vi "NOAH_jr.vi"() -> ()   [LabVIEW 2017]
panel:
  in  "Rates":dbl
  in  "Outliers":dbl
  in  "Max":dbl
  in  "Min":dbl
  in  "Range":dbl
  in  "Standard Deviation":dbl
  in  "Median":dbl
  in  "Mean":dbl
  in  "Data Source":string
  in  "Fault Text":string
  out "Posting Time":timestamp format="%<%H:%M:%S>T"
  out "Time to Handle":timestamp format="%<%H:%M:%S>T"
  out "Fault Priority Rank":dbl
  out "Notification Light":bool
  out "OK Time":timestamp format="%<%H:%M:%S>T"
  in  "Problem Count":dbl
  in  "Prompt Count":dbl
  in  "Warning Count":dbl
  in  "Total Notifications":dbl format="%#.0g"
  # "At-a-Glance"
  # "Fault Information"
  # "Priority"
  # "to handle"
  # "Posted at"
  # "Pinned Items"
  # "Analytics"
  # "Model HQ"
  # "Analytical"
  # "Grey-Box"
  # "Data-Driven"
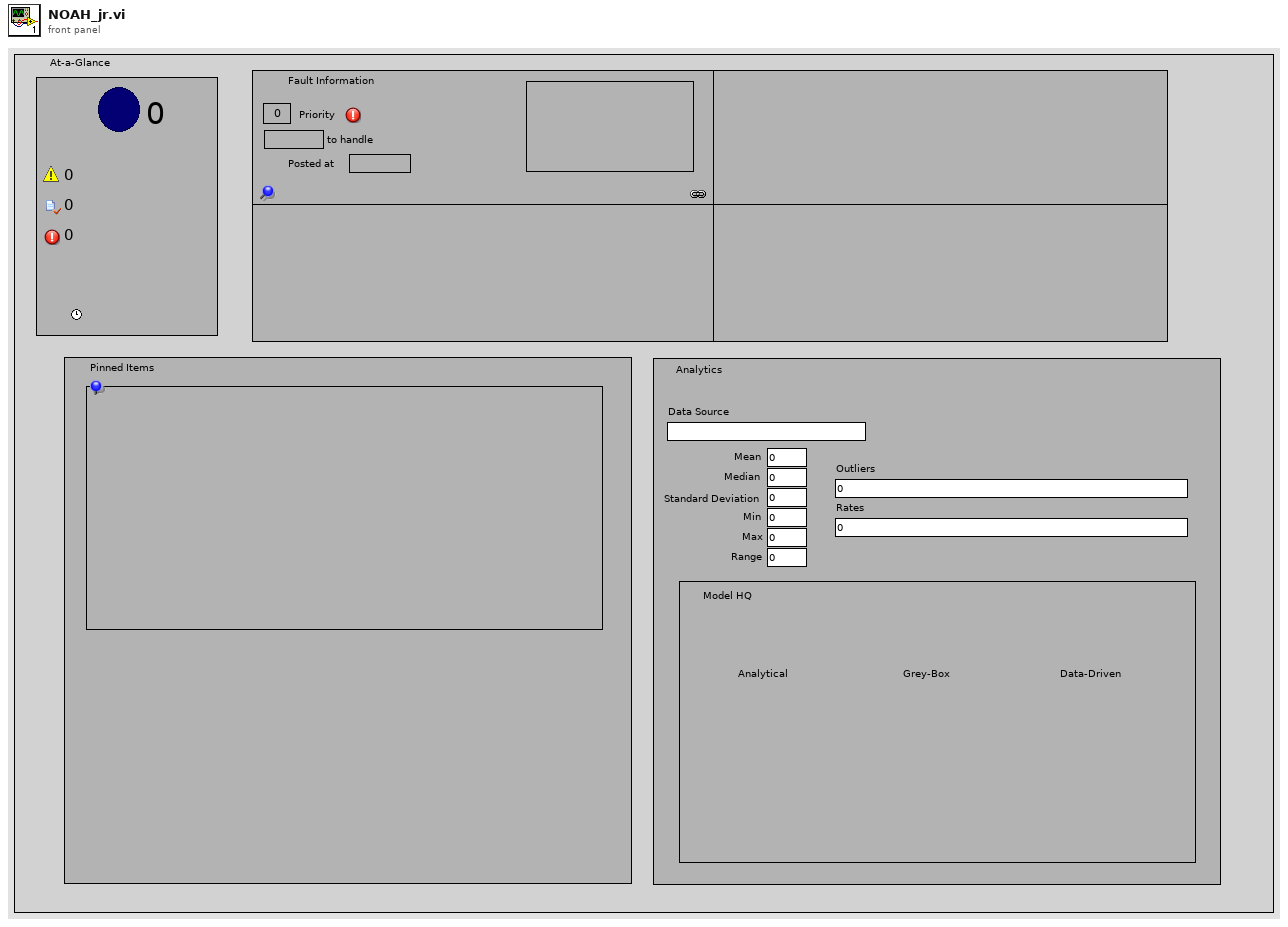
[diagram p1: front panel]
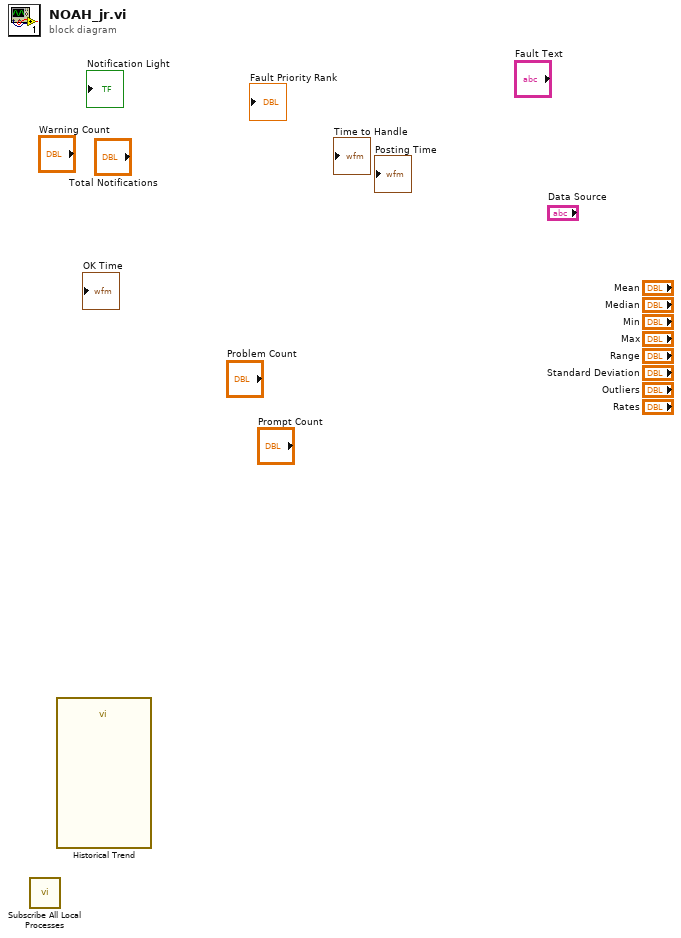
[diagram p0: block diagram]
diagram:
  n1 = call <vilib>:"Subscribe All Local Processes.vi"() -> ("Alarm & Event Displayer reference"=w1:refnum<k7>)  [unwired: 9 in, 2 out]
  n2 = call "Historical Trend"() -> ()  [unwired: 8 in, 4 out]
